vi "prova.vi"() -> ()   [LabVIEW 2025]
uses:
  <instrlib>/Keithley 2600 Series/Keithley 2600 Series.lvlib
panel:
  out "String 5":string
  out "String 4":string
  out "String 3":string
  out "String 2":string
  out "range misurato":string
  out "range misurato 2":string
  in  "source_range_gate":dbl format="%#_13g"
  in  "source_range_drain":dbl format="%#_13g"
  in  "dual sweep":bool
  out "error out":errorcluster
  in  "Boolean 4":bool
  in  "Boolean 3":bool
  in  "inverti smu":bool
  in  "Autozero Mode (2: Autozero Auto) 2":i32(ring)=2 items=["Autozero Off", "Autozero Once", "Autozero Auto"]
  in  "Autozero Mode (2: Autozero Auto)":i32(ring)=2 items=["Autozero Off", "Autozero Once", "Autozero Auto"]
  in  "Source Function (1: Voltage) 2":i32(ring)=1 items=["Current", "Voltage"]
  in  "Range Mode (1: Auto Range On) 2":i32(ring)=1 items=["Auto Range Off", "Auto Range On", "Auto Range Follow Limit"]
  in  "Source Function (1: Voltage)":i32(ring)=1 items=["Current", "Voltage"]
  in  "Range Mode (1: Auto Range On)":i32(ring)=1 items=["Auto Range Off", "Auto Range On", "Auto Range Follow Limit"]
  in  "range-gate":dbl format="%#_13g"
  in  "range-drain":dbl format="%#_13g"
  in  "limit-gate":dbl format="%#_13g"
  in  "limit-drain":dbl format="%#_13g"
  out "intervallo tra due misure approx (S)":dbl
  out "Frequenza di rete (Hz)":dbl
  in  "Numero di punti":i32
  out "finestra di misura (S)":dbl
  in  "Delay Time (S)":dbl
  in  "String":string
  in  "numero di sweep ripetute\n(piramidi per dual sweep)":i32
  in  "nplc":dbl
  in  "Boolean":bool
  in  "Pulse Stop Level (1 V) 2":dbl
  in  "Pulse Start Level (0 V) 2":dbl
  out "SMUB-TEMPI":dbl[](array[numeric])
  out "SMUB-TENSIONE":dbl[](array[numeric])
  out "SMUB-CORRENTE":dbl[](array[numeric])
  out "SMUA-TEMPI":dbl[](array[numeric])
  out "SMUA-TENSIONE":dbl[](array[numeric])
  out "SMUA-CORRENTE":dbl[](array[numeric])
  in  "stop 2":bool
  in  "stop":bool
  out "Firmware Revision":string
  out "Serial Number":string
  out "Model":string
  in  "VISA resource name":refnum<visa-resource-name>
  # "Impostazioni funzione source"
  # "Impostazioni connessione"
  # "DRAIN"
  # "GATE"
  # "Auto Range Off"
  # "Auto Range On"
  # "Auto Range Off"
  # "Auto Range On"
  # "non utilizzato...funzioni di lua per automatizzare il range"
  # "Impostazioni comuni"
  # "Impostazioni funzione misura"
  # "GATE"
  # "DRAIN"
  # "(1/"
  # "X"
  # ")"
  # "Auto Range Off"
  # "Auto Range On"
  # "Auto Range Off"
  # "Auto Range On"
  # "+"
  # "Controllo misura"
  # "tabella valori"
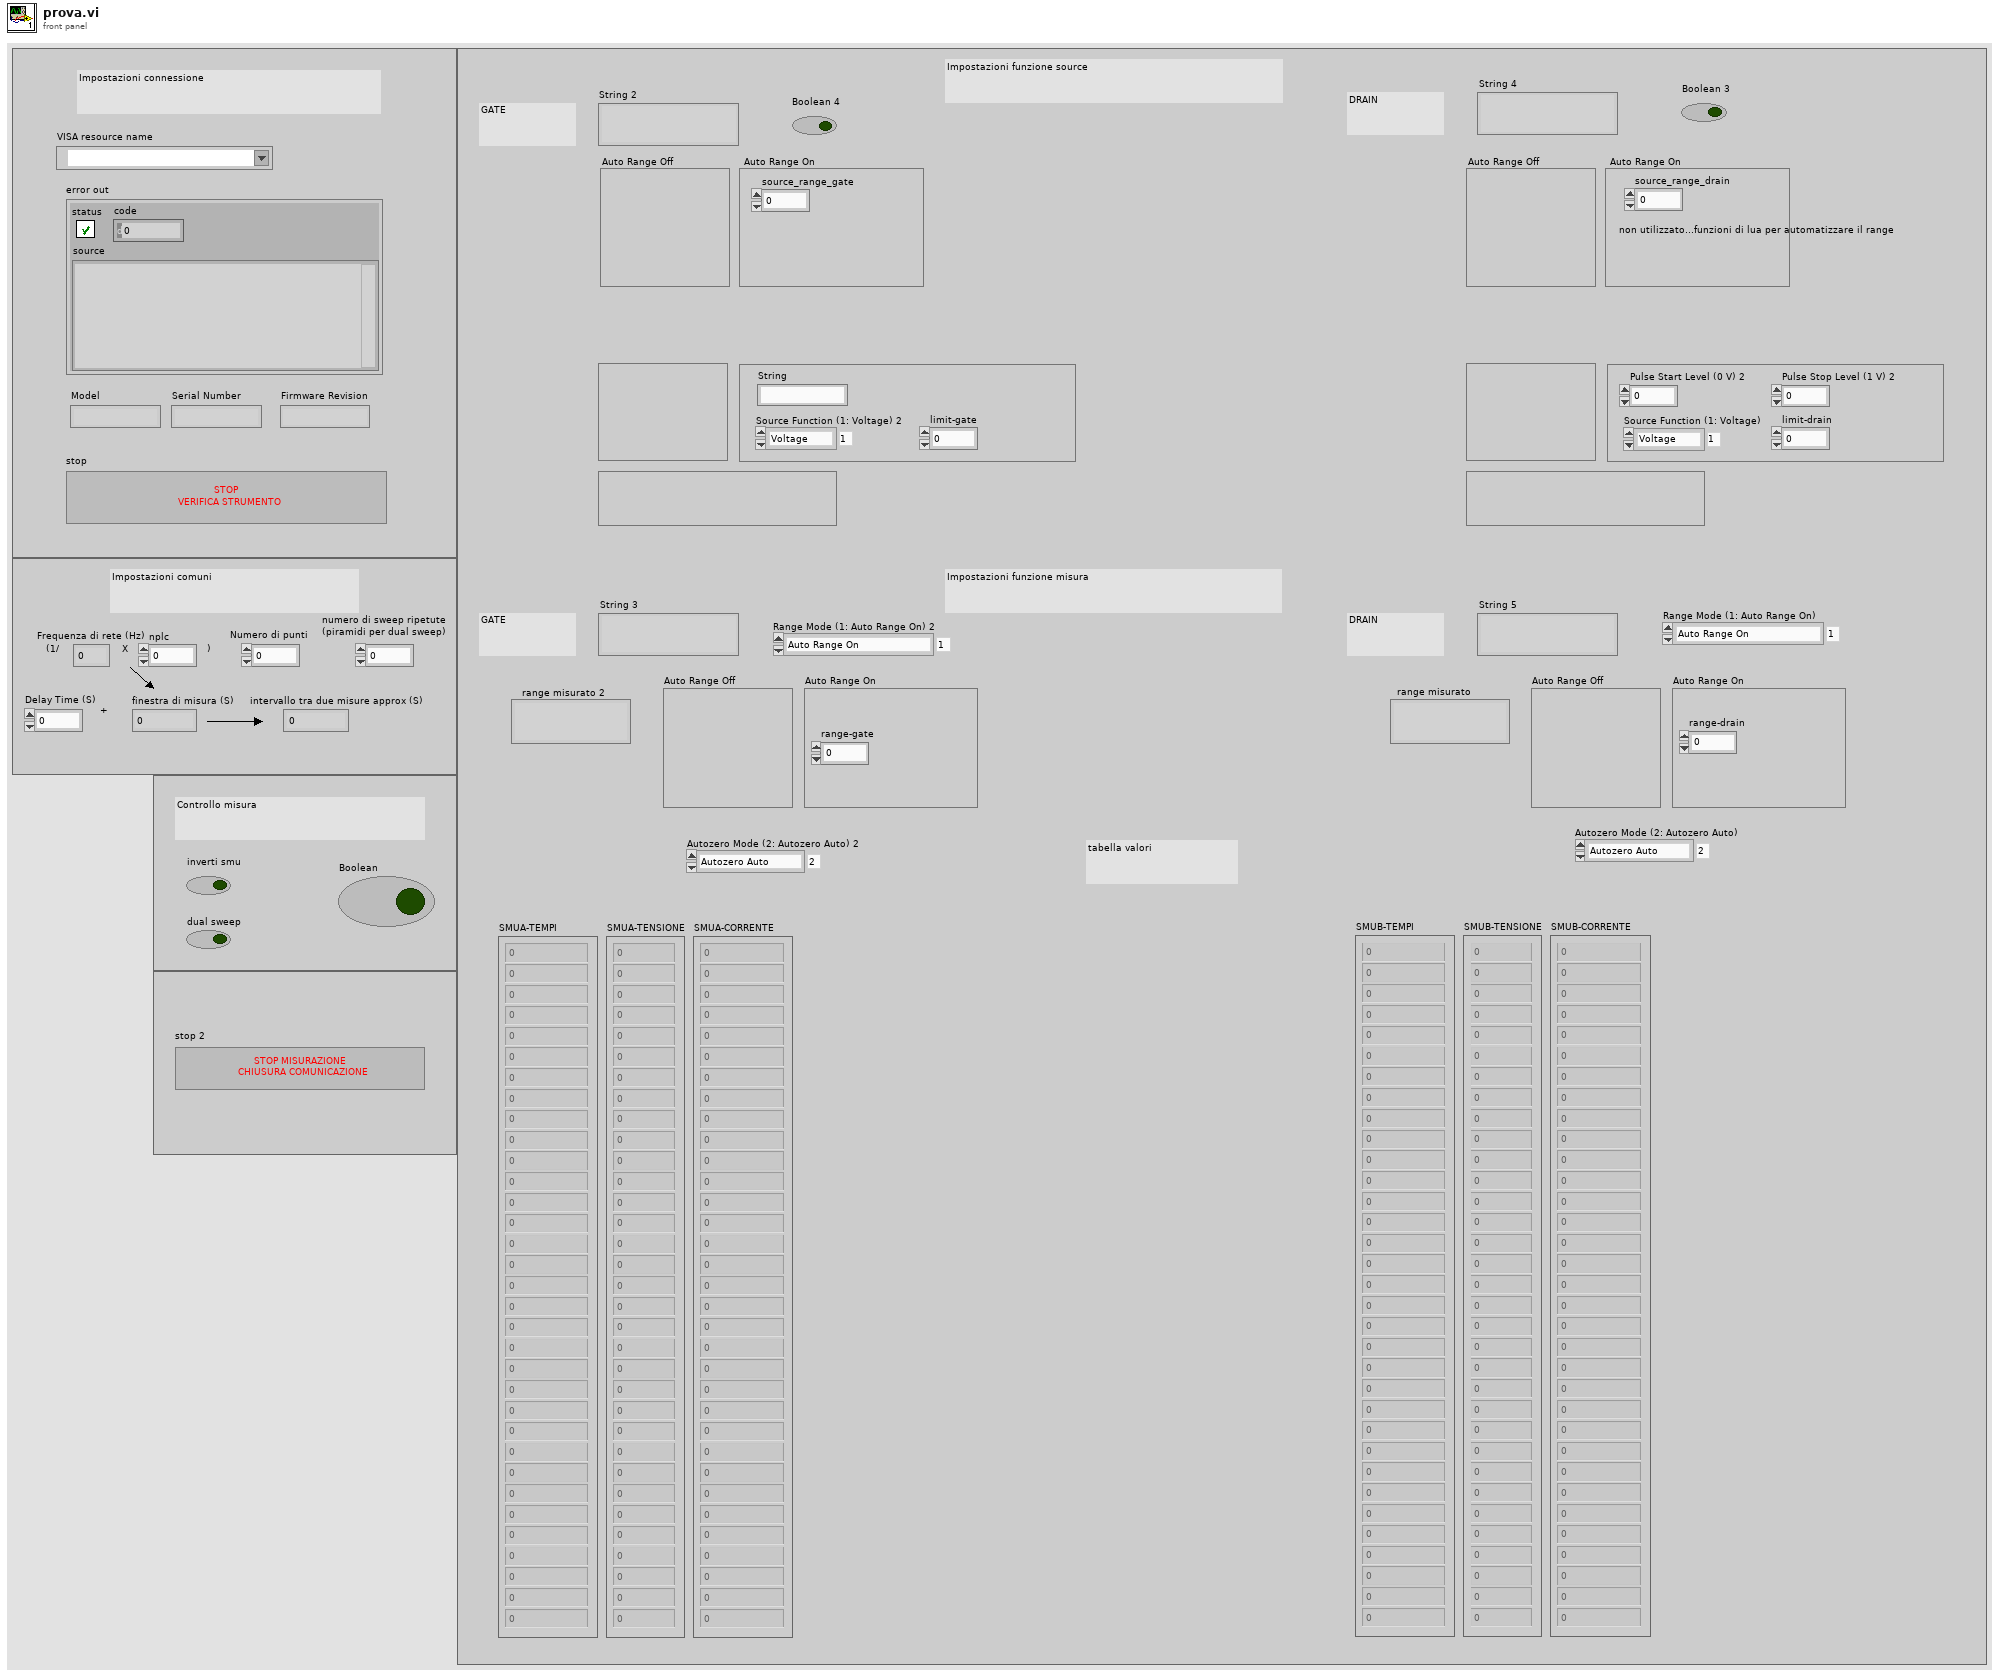
[diagram p1: front panel]
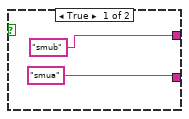
[diagram p2: hidden frame]
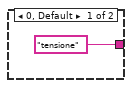
[diagram p3: hidden frame]
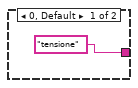
[diagram p4: hidden frame]
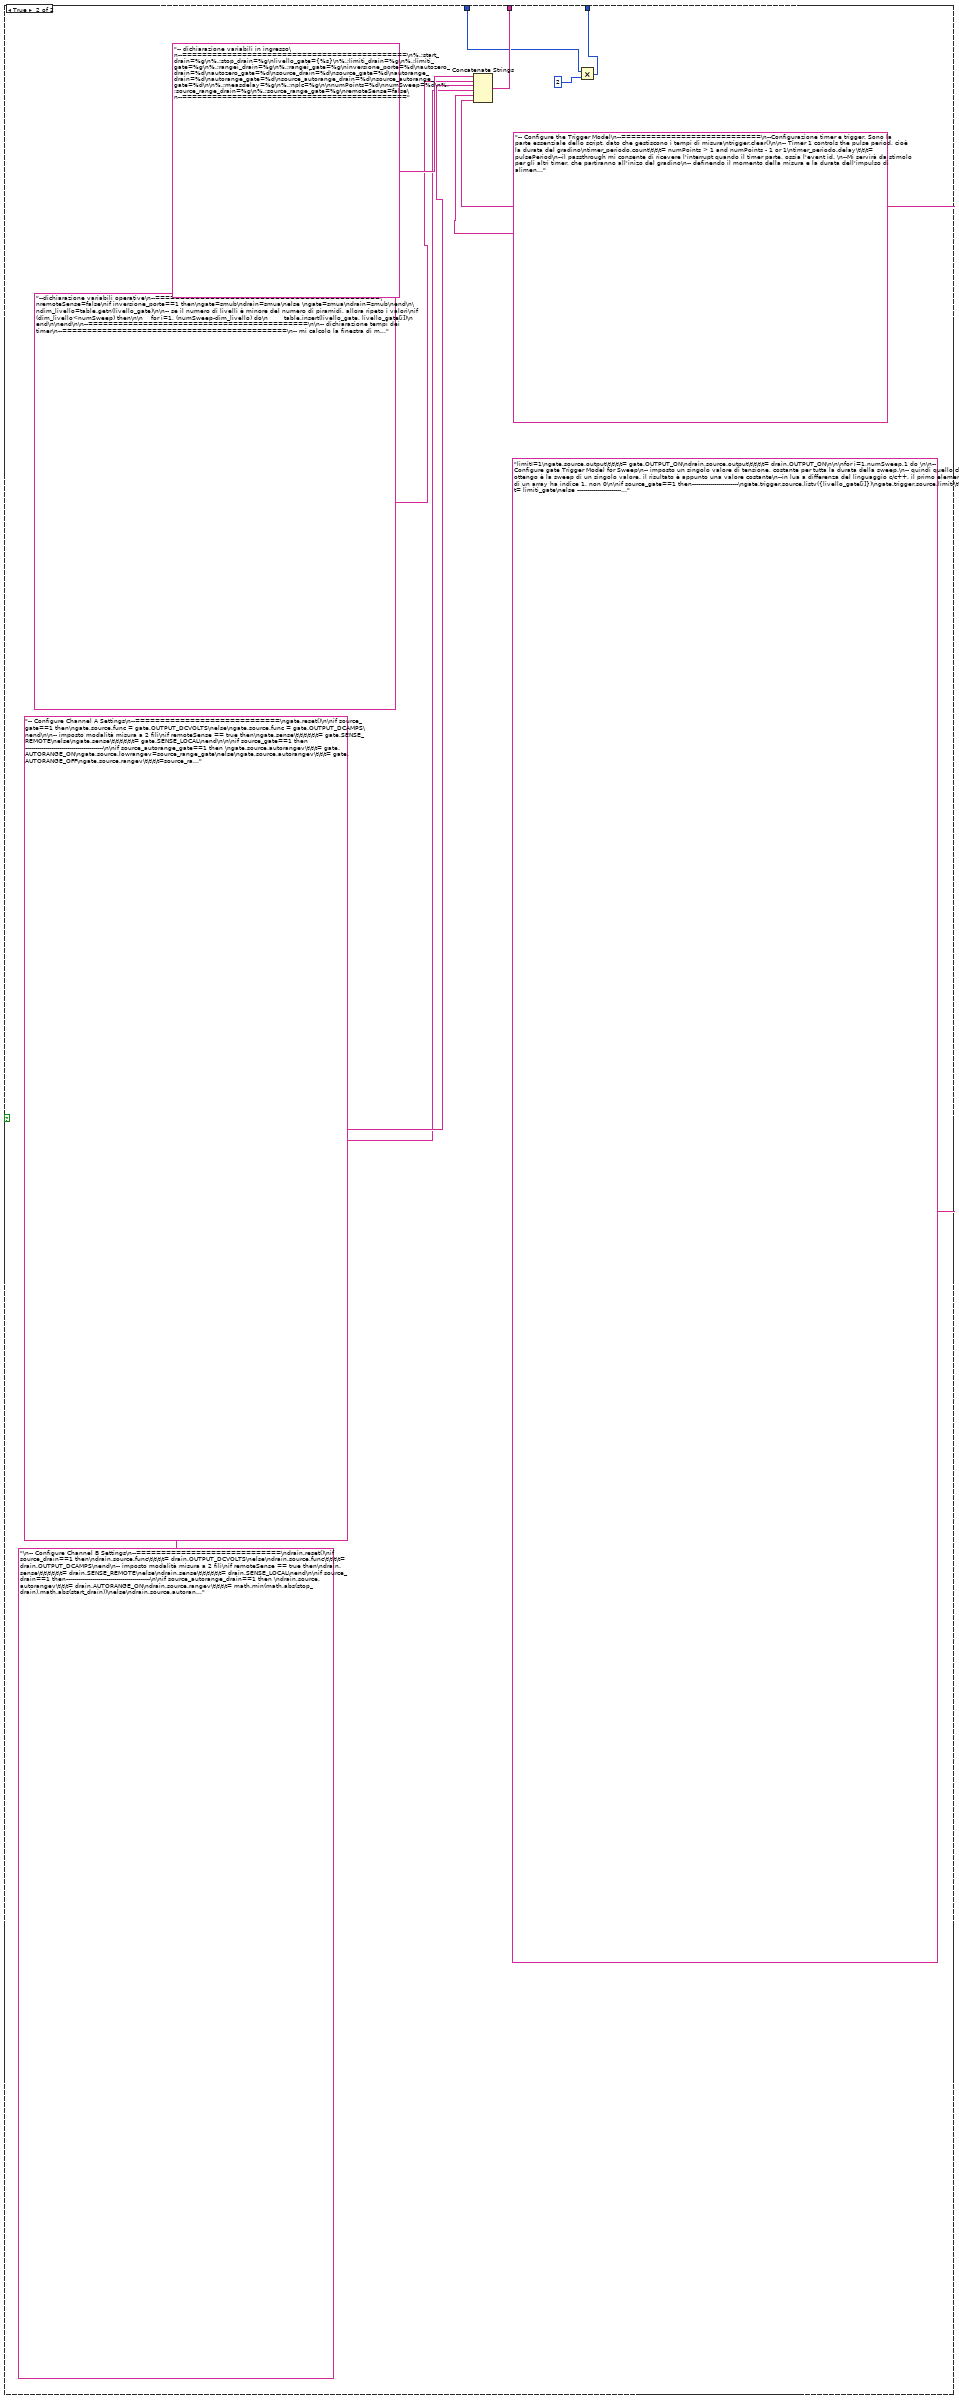
[diagram p6: hidden frame]
diagram:
  n1 = flat-sequence {
    tunnel: [w10] -> w5
    tunnel: [w7] -> w4
    tunnel: [w14] -> w6
    tunnel: w5 -> [w16]
    tunnel: w4 -> [w15]
    tunnel: [w13] -> w3
    tunnel: w6 -> [w28]
    tunnel: w3 -> [w27]
    tunnel: [w26] -> w2
    tunnel: [w25] -> w1
    tunnel: w2 -> [w147]
    tunnel: w1 -> [w146]
    frame #0 {
      w11 = "0\n\n"
      n2 = local write "Firmware Revision"(w11) -> ()
      n3 = local write "Serial Number"(w11) -> ()
      n4 = local write "Model"(w11) -> ()
      n5 = call <instrlib>:"Initialize.vi"("Reset (True)"=TRUE, "ID Query (True)"=FALSE, "VISA resource name"="VISA resource name") -> ("error out"=w7:errorcluster, "VISA resource name out"=w10:refnum<visa-resource-name>)  [unwired: 7 in]
      "error out" <- w7
    }
    frame #1 {
      n6 = while {
        tunnel: w16 -> [w20]
        tunnel: w15 -> [w19]
        tunnel: [w18] -> w14
        tunnel: [w17] -> w13
        stop <- "stop" stop-if-true
        n7 = call <instrlib>:"Query Local Node Identity.vi"("error in (no error)"=w19, "VISA resource name"=w20) -> ("error out"=w17:errorcluster, "Serial Number"=→"Serial Number":string, "Model"=→"Model":string, "VISA resource name out"=w18:refnum<visa-resource-name>, "Firmware Revision"=→"Firmware Revision":string)  [unwired: 5 in]
      }
    }
    frame #2 {
      n8 = while {
        tunnel: w28 -> [w53]
        tunnel: w27 -> [w52]
        tunnel: [w68] -> w26
        tunnel: [w67] -> w25
        stop <- "stop 2" stop-if-true
        n9 = case shown="False" "inverti smu" {
          tunnel: ["smub" "smua"] -> w31
          tunnel: ["smua" "smub"] -> w30
          frame True {
          }
          frame False {
          }
        }
        "String 2" <- w31
        "String 3" <- w31
        "String 4" <- w30
        "String 5" <- w30
        n10 = call <instrlib>:"Print Variable.vi"("error in (no error)"=w52, "Variable Name"="localnode.linefreq", "VISA resource name"=w53) -> ("error out"=w50:errorcluster, "Number"=w57:dbl, "VISA resource name out"=w51:refnum<visa-resource-name>)  [unwired: 5 in, 1 out]
        "Frequenza di rete (Hz)" <- w57
        n11 = Divide(x=1.0, y=w57) -> (x/y=w62:dbl)
        n12 = Multiply(x="nplc", y=w62) -> (x*y=w54:dbl)
        "finestra di misura (S)" <- w54
        n13 = Add(x="Delay Time (S)", y=w54) -> (x+y=→"intervallo tra due misure approx (S)":dbl)
        n14 = case shown="1" "Source Function (1: Voltage) 2" {
          tunnel: ["tensione" "corrente"] -> w34
          frame 0, Default {
          }
          frame 1 {
          }
        }
        "range misurato" <- w34
        n15 = case shown="1" "Source Function (1: Voltage)" {
          tunnel: ["tensione" "corrente"] -> w35
          frame 0, Default {
          }
          frame 1 {
          }
        }
        "range misurato 2" <- w35
        n16 = case shown="True" "Boolean" {
          tunnel: [w79 w114] -> w68
          tunnel: [w78 w113] -> w67
          tunnel: w50 -> [w78 w123]
          tunnel: w51 -> [w79 w124]
          tunnel: "Pulse Start Level (0 V) 2" -> [_ w104]
          tunnel: "Pulse Stop Level (1 V) 2" -> [_ w103]
          tunnel: "Numero di punti" -> [_ w85]
          tunnel: "Delay Time (S)" -> [_ w89]
          tunnel: "numero di sweep ripetute\n(piramidi per dual sweep)" -> [_ w84]
          tunnel: "String" -> [_ w102]
          tunnel: "limit-drain" -> [_ w101]
          tunnel: "limit-gate" -> [_ w100]
          tunnel: "range-drain" -> [_ w99]
          tunnel: "range-gate" -> [_ w98]
          tunnel: "inverti smu" -> [_ w97]
          tunnel: "Autozero Mode (2: Autozero Auto)" -> [_ w96]
          tunnel: "Autozero Mode (2: Autozero Auto) 2" -> [_ w95]
          tunnel: "Source Function (1: Voltage)" -> [_ w94]
          tunnel: "Source Function (1: Voltage) 2" -> [_ w93]
          tunnel: "Range Mode (1: Auto Range On)" -> [_ w92]
          tunnel: "Range Mode (1: Auto Range On) 2" -> [_ w91]
          tunnel: "nplc" -> [_ w90]
          tunnel: "Boolean 3" -> [_ w88]
          tunnel: "Boolean 4" -> [_ w87]
          tunnel: "dual sweep" -> [_ w86]
          tunnel: "source_range_drain" -> [_ w81]
          tunnel: "source_range_gate" -> [_ w80]
          frame False {
          }
          frame True {
            w112 = 0 items=["Channel A", "Channel B"] ("Source Measure Unit Channel (0: Channel A)")
            w115 = 1 items=["Channel A", "Channel B"] ("Source Measure Unit Channel (0: Channel A)")
            n17 = Multiply(x=w85, y=w84) -> (x*y=w83:i32)
            n18 = case shown="False" w86 {
              tunnel: [w128 w139] -> w105
              tunnel: w83 -> [w127 w137]
              tunnel: [w126 w138] -> w82
              frame False {
                n19 = Concatenate Strings("-- dichiarazione variabili in ingresso\n--=============================================\n%.;start_drain=%g\n%.;stop_drain=%g\nlivello_gate={%s}\n%.;limiti_drain=%g\n%.;limiti_gate=%g\n%.;rangei_drain=%g\n%.;rangei_gate=%g\ninversione_porte=%d\nautozero_drain=%d\nautozero_gate=%d\nsource_drain=%d\nsource_gate=%d\nautorange_drain=%d\nautorange_gate=%d\nsource_autorange_drain=%d\nsource_autorange_gate=%d\n\n%.;measdelay=%g\n%.;nplc=%g\n\nnumPoints=%d\nnumSweep=%d\nremoteSense=false\n%.;source_range_drain=%g\n%.;source_range_gate=%g\n--=============================================", "--dichiarazione variabili operative\n--=============================================\nremoteSense=false\nif inversione_porte==1 then\ngate=smub\ndrain=smua\nelse \ngate=smua\ndrain=smub\nend\n--============================================\n\n-- dichiarazione tempi dei timer\n--=============================================\n-- mi calcolo la finestra di misura\nfinestra_misura=(1/localnode.linefreq)*nplc\n-- imposto la lunghezza dell'impulso. la dc sweep si origina da una pulsed sweep.\npulseWidth=measdelay+finestra_misura \n--il periodo è l'impulso + più un t_off, una bassa percentuale dell'impulso\npulsePeriod=pulseWidth+(pulseWidth*1/100) \n\n--=============================================\n\n-- dichiarazione timer e gestore eventi\n--=============================================\n-- Timer 1: timer periodo (larghezza gradino)\ntimer_periodo=trigger.timer[1]\n-- Timer 2: Timer ritardo misura\ntimer_misura=trigger.timer[2]\n-- Timer 3: Pulse Width Timer\ntimer_larghezza_impulso=trigger.timer[3]\n\n-- Gestore eventi 1: Event Blender per la partenza di iniziale di smua e l'aggiornamento di smua al trigger di smub\ngestore_avvio_gate=trigger.blender[1]\n--=============================================", "-- Configure Channel A Settings\n--=============================\ngate.reset()\n\nif source_gate==1 then\ngate.source.func = gate.OUTPUT_DCVOLTS\nelse\ngate.source.func = gate.OUTPUT_DCAMPS\nend\n\n-- imposto modalità misura a 2 fili\nif remoteSense == true then\ngate.sense\t\t\t\t\t\t= gate.SENSE_REMOTE\nelse\ngate.sense\t\t\t\t\t\t= gate.SENSE_LOCAL\nend\n\n\nif source_gate==1 then ---------------------------------------\n\nif source_autorange_gate==1 then \ngate.source.autorangev\t\t\t= gate.AUTORANGE_ON\ngate.source.lowrangev= source_range_gate\nelse\ngate.source.autorangev\t\t\t= gate.AUTORANGE_OFF\ngate.source.rangev\t\t\t\t= source_range_gate\nend \n\ngate.source.levelv\t\t\t\t= 0\n-- Set the DC bias limit.  This is not the limit used during the pulses. ma è il valore di idle della gate\ngate.source.limiti\t\t\t\t= limiti_gate\n\nelse------------------------\n\nif source_autorange_gate==1 then\ngate.source.autorangei\t\t\t= gate.AUTORANGE_ON\ngate.source.lowrangei=source_range_gate\nelse\ngate.source.autorangei\t\t\t= gate.AUTORANGE_OFF\ngate.source.rangei\t\t\t=source_range_gate\nend\n\ngate.source.leveli\t\t\t\t= 0\n-- Set the DC bias limit.  This is not the limit used during the pulses. ma è il valore di idle della gate\ngate.source.limitv\t\t\t\t= limiti_gate\nend --------------------------------------------------\n\n\n-- Disabling Auto-Ranging and Auto-Zero ensures accurate and consistent timing\nif autozero_gate==0 then\ngate.measure.autozero\t\t\t= gate.AUTOZERO_OFF\nelseif autozero_gate==1 then\ngate.measure.autozero\t\t\t= gate.AUTOZERO_ONCE\nelse\ngate.measure.autozero\t\t\t= gate.AUTOZERO_AUTO\nend\n\nif autorange_gate==0 then ------------------------\n\nif source_gate==1 then\ngate.measure.autorangei\t\t\t= gate.AUTORANGE_OFF\ngate.measure.rangei\t\t\t\t= rangei_gate\nelse\ngate.measure.autorangev\t\t\t= gate.AUTORANGE_OFF\ngate.measure.rangev\t\t\t\t= rangei_gate\nend\n\nelseif  autorange_gate==1 then -----------\n\nif source_gate==1 then\ngate.measure.autorangei\t\t\t= gate.AUTORANGE_ON\ngate.measure.lowrangei\t\t\t\t= rangei_gate\nelse\ngate.measure.autorangev\t\t\t= gate.AUTORANGE_ON\ngate.measure.lowrangev\t\t\t\t= rangei_gate\nend\n\nelse --------------------------\n\nend -------------------------------\n\ngate.measure.nplc\t\t\t\t= nplc\n-- A timer will be used to set the measure delay and synchronize the measurement\n-- between the two SMUs so set the built in delay to 0.\ngate.measure.delay\t\t\t\t= 0\n\n-- Prepare the Reading Buffers\ngate.nvbuffer1.clear()\ngate.nvbuffer1.collecttimestamps= 1\ngate.nvbuffer2.clear()\ngate.nvbuffer2.collecttimestamps = 1\n--=============================\n-- End Channel A Settings", "\n-- Configure Channel B Settings\n--=============================\ndrain.reset()\nif source_drain==1 then\ndrain.source.func\t\t\t\t= drain.OUTPUT_DCVOLTS\nelse\ndrain.source.func\t\t\t\t= drain.OUTPUT_DCAMPS\nend\n-- imposto modalità misura a 2 fili\nif remoteSense == true then\ndrain.sense\t\t\t\t\t\t= drain.SENSE_REMOTE\nelse\ndrain.sense\t\t\t\t\t\t= drain.SENSE_LOCAL\nend\n\nif source_drain==1 then------------------------------------------\n\nif source_autorange_drain==1 then \ndrain.source.autorangev\t\t\t= drain.AUTORANGE_ON\ndrain.source.rangev\t\t\t\t= math.min(math.abs(stop_drain),math.abs(start_drain))\nelse\ndrain.source.autorangev\t\t\t= drain.AUTORANGE_OFF\ndrain.source.rangev\t\t\t\t=  math.max(math.abs(stop_drain),math.abs(start_drain))\nend\n\ndrain.source.levelv\t\t\t\t= 0\n-- Set the DC bias limit.  This is not the limit used during the pulses. ma è il valore di idle della smu\ndrain.source.limiti\t\t\t\t= limiti_drain\nelse----------------------------------------------------\nif source_autorange_drain==1 then \ndrain.source.autorangei\t\t\t= drain.AUTORANGE_ON\ndrain.source.rangei\t\t\t\t= math.min(math.abs(stop_drain),math.abs(start_drain))\nelse\ndrain.source.autorangei\t\t\t= drain.AUTORANGE_OFF\ndrain.source.rangei\t\t\t\t= math.max(math.abs(stop_drain),math.abs(start_drain))\nend\ndrain.source.leveli\t\t\t\t= 0\n-- Set the DC bias limit.  This is not the limit used during the pulses. ma è il valore di idle della smu\ndrain.source.limitv\t\t\t\t= limiti_drain\nend----------------------------------------------\n\n-- Disabling Auto-Ranging and Auto-Zero ensures accurate and consistent timing\n\nif autozero_drain==0 then\ndrain.measure.autozero\t\t\t= drain.AUTOZERO_OFF\nelseif autozero_drain==1 then\ndrain.measure.autozero\t\t\t= drain.AUTOZERO_ONCE\nelseif autozero_drain==2 then\ndrain.measure.autozero\t\t\t= drain.AUTOZERO_AUTO\nend\n\nif autorange_drain==0 then --------------------------------\n\nif source_drain==1 then\ndrain.measure.autorangei\t\t\t= drain.AUTORANGE_OFF\ndrain.measure.rangei\t\t\t\t= rangei_drain\nelse\ndrain.measure.autorangev\t\t\t= drain.AUTORANGE_OFF\ndrain.measure.rangev\t\t\t\t= rangei_drain\nend\n\n\n\nelseif  autorange_drain==1 then ----------------------------\n\nif source_drain==1 then\ndrain.measure.autorangei\t\t\t= drain.AUTORANGE_ON\ndrain.measure.lowrangei\t\t\t\t= rangei_drain\nelse\ndrain.measure.autorangev\t\t\t= drain.AUTORANGE_ON\ndrain.measure.lowrangev\t\t\t\t= rangei_drain\nend\n\nelse\n\nend --------------------------------------------------------------\n\ndrain.measure.nplc\t\t\t\t= nplc\n-- A timer will be used to set the measure delay and synchronize the measurement\n-- between the two SMUs so set the built in delay to 0.\ndrain.measure.delay\t\t\t\t= 0\n\n-- Prepare the Reading Buffers\ndrain.nvbuffer1.clear()\ndrain.nvbuffer1.collecttimestamps= 1\ndrain.nvbuffer2.clear()\ndrain.nvbuffer2.collecttimestamps= 1\n--=============================\n-- End Channel B Settings", "-- Configure the Trigger Model\n--============================\n--Configurazione timer e trigger. Sono la parte essenziale dello script, dato che gestiscono i tempi di misura\ntrigger.clear()\n\n-- Timer 1 controls the pulse period, cioè la durata del gradino\ntimer_periodo.count\t\t\t= numPoints > 1 and numPoints - 1 or 1\ntimer_periodo.delay\t\t\t= pulsePeriod\n--il passthrough mi consente di ricevere l'interrupt quando il timer parte, ossia l'event id. \n--Mi servirà da stimolo per gli altri timer, che partiranno all'inizo del gradino\n-- definendo il momento della misura e la durata dell'impulso di alimentazione\ntimer_periodo.passthrough\t= true\n-- il timer 1 parte quando la drain, in questo caso, inizia la sweep: cioè entra nello stato armed\ntimer_periodo.stimulus\t\t= drain.trigger.ARMED_EVENT_ID \n\n-- Timer 2 controls the measurement. il timer 2 gestisce il ritardo di misura. scaduto quello, inizia la finestra di misura\ntimer_misura.count\t\t\t= 1\ntimer_misura.delay\t\t\t= measdelay\n-- il passthrough è false perchè l'interrupt lo produrre alla fine. \n-- Scaduto il delay di misura, inizia la finestra di misura\ntimer_misura.passthrough\t= false\n--il timer 1 grazie al passthrough mi fa partire il timer 2 all'inizio del gradino\ntimer_misura.stimulus\t\t= timer_periodo.EVENT_ID \n\n-- Timer 3 controls the pulse width\ntimer_larghezza_impulso.count\t\t\t= 1\ntimer_larghezza_impulso.delay\t\t\t= pulseWidth\n-- il passthrough è false perchè l'interrupt me lo produce alla fine, perchè \ntimer_larghezza_impulso.passthrough\t= false\n--il timer 1 grazie al passthrough mi fa partire il timer 3 all'inizio del gradino\ntimer_larghezza_impulso.stimulus\t\t= timer_periodo.EVENT_ID\n", "\n-- Configure gate Trigger Model for Sweep\n-- imposto un singolo valore di tensione, costante per tutta la durata della sweep.\n-- quindi quello che ottengo è la sweep di un singolo valore. il risultato è appunto una valore costante\nif source_gate==1 then-----------------------\ngate.trigger.source.listv(livello_gate)\ngate.trigger.source.limiti\t\t= limiti_gate\nelse -------------------------------------------\ngate.trigger.source.listi(livello_gate)\ngate.trigger.source.limitv\t\t= limiti_gate\nend--------------------------------------------\ngate.trigger.measure.action\t\t= gate.ASYNC\ngate.trigger.measure.iv(gate.nvbuffer1, gate.nvbuffer2)\n--fine impulso: se voglio una dc sweep, anzichè mandare in idle l'uscita, la tengo costante\ngate.trigger.endpulse.action\t= gate.SOURCE_HOLD\n-- endsweep mi dice cosa fare quando finisce l'operazione sweep\ngate.trigger.endsweep.action\t= gate.SOURCE_HOLD\ngate.trigger.arm.count = 1\ngate.trigger.count\t\t\t\t= numSweep\n-- arm sweep indica quanto sweep deve fare \ndrain.trigger.arm.stimulus\t\t= 0\n\n\n--event blender per la partenza\ngestore_avvio_gate.orenable = true\ngestore_avvio_gate.stimulus[1] = gate.trigger.ARMED_EVENT_ID\ngestore_avvio_gate.stimulus[2] = drain.trigger.ARMED_EVENT_ID \n\n--dico quali stimoli/timer attivano le azioni\ngate.trigger.source.stimulus = gestore_avvio_gate.EVENT_ID \ngate.trigger.measure.stimulus\t= timer_misura.EVENT_ID\ngate.trigger.endpulse.stimulus\t= drain.trigger.SWEEP_COMPLETE_EVENT_ID\n\ngate.trigger.source.action\t\t= gate.ENABLE\n\n-- Configure drain Trigger Model for Sweep\nif source_drain==1 then------------------------\ndrain.trigger.source.linearv(start_drain, stop_drain, numPoints)\ndrain.trigger.source.limiti\t\t= limiti_drain\nelse---------------------------------------------\ndrain.trigger.source.lineari(start_drain, stop_drain, numPoints)\ndrain.trigger.source.limitv\t\t= limiti_drain\nend---------------------------------------------\ndrain.trigger.measure.action\t\t= drain.ENABLE\ndrain.trigger.measure.iv(drain.nvbuffer1, drain.nvbuffer2)\n--fine impulso: se voglio una dc sweep, anzichè mandare in idle l'uscita, la tengo costante\ndrain.trigger.endpulse.action\t= drain.SOURCE_HOLD \n-- endsweep mi dice cosa fare quando finisce l'operazione sweep\ndrain.trigger.endsweep.action\t= drain.SOURCE_HOLD\ndrain.trigger.arm.count = numSweep\n-- num punti sweep\ndrain.trigger.count\t\t\t\t= numPoints\n-- arm sweep indica quanto sweep deve fare\ndrain.trigger.arm.stimulus\t\t= 0\n--dico quali timer attivanzo le azioni\ndrain.trigger.source.stimulus\t= timer_periodo.EVENT_ID\ndrain.trigger.measure.stimulus\t= timer_misura.EVENT_ID\ndrain.trigger.endpulse.stimulus\t= timer_larghezza_impulso.EVENT_ID\ndrain.trigger.source.action\t\t= drain.ENABLE\n--==============================\n-- End Trigger Model Configuration" ("write buffer"), "\ngate.source.output\t\t\t\t= gate.OUTPUT_ON\ndrain.source.output\t\t\t\t= drain.OUTPUT_ON\n\n-- Start the trigger model execution\ngate.trigger.initiate()\ndelay(0.05)\ndrain.trigger.initiate()\n\n-- Wait until the sweep has completed\nwaitcomplete()\n\ndrain.source.output\t\t\t\t= drain.OUTPUT_OFF\ndelay(0.05)\ngate.source.output\t\t\t\t= gate.OUTPUT_OFF\n\n--printbuffer(1, numPoints, gate.nvbuffer2.readings)\n--printbuffer(1, numPoints, gate.nvbuffer1.readings)\n--printbuffer(1, numPoints, gate.nvbuffer1.timestamps)\n\n--printbuffer(1, numPoints, drain.nvbuffer2.readings)\n--printbuffer(1, numPoints, drain.nvbuffer1.readings)\n--printbuffer(1, numPoints, drain.nvbuffer1.timestamps)\n") -> (w128:string)
                n20 = Multiply(x=w127, y=1) -> (x*y=w126:i32)
              }
              frame True {
                n21 = Concatenate Strings("-- dichiarazione variabili in ingresso\n--=============================================\n%.;start_drain=%g\n%.;stop_drain=%g\nlivello_gate={%s}\n%.;limiti_drain=%g\n%.;limiti_gate=%g\n%.;rangei_drain=%g\n%.;rangei_gate=%g\ninversione_porte=%d\nautozero_drain=%d\nautozero_gate=%d\nsource_drain=%d\nsource_gate=%d\nautorange_drain=%d\nautorange_gate=%d\nsource_autorange_drain=%d\nsource_autorange_gate=%d\n\n%.;measdelay=%g\n%.;nplc=%g\n\nnumPoints=%d\nnumSweep=%d\n%.;source_range_drain=%g\n%.;source_range_gate=%g\nremoteSense=false\n--=============================================", "--dichiarazione variabili operative\n--=============================================\nremoteSense=false\nif inversione_porte==1 then\ngate=smub\ndrain=smua\nelse \ngate=smua\ndrain=smub\nend\n\ndim_livello=table.getn(livello_gate)\n\n-- se il numero di livelli è minore del numero di piramidi, allora ripeto i valori\nif (dim_livello<numSweep) then\n\n    for i=1, (numSweep-dim_livello) do\n        table.insert(livello_gate, livello_gate[i])\n    end\n\nend\n\n--============================================\n\n-- dichiarazione tempi dei timer\n--=============================================\n-- mi calcolo la finestra di misura\nfinestra_misura=(1/localnode.linefreq)*nplc\n-- imposto la lunghezza dell'impulso. la dc sweep si origina da una pulsed sweep.\npulseWidth=measdelay+finestra_misura \n--il periodo è l'impulso + più un t_off, una bassa percentuale dell'impulso\npulsePeriod=pulseWidth+(pulseWidth*1/100) \n--=============================================\n\n-- dichiarazione timer e gestore eventi\n--=============================================\n-- Timer 1: timer periodo (larghezza gradino)\ntimer_periodo=trigger.timer[1]\n-- Timer 2: Timer ritardo misura\ntimer_misura=trigger.timer[2]\n-- Timer 3: Pulse Width Timer\ntimer_larghezza_impulso=trigger.timer[3]\n\n-- Gestore eventi 1: Event Blender per la partenza di iniziale di smua e l'aggiornamento di smua al trigger di smub\ngestore_avvio_gate=trigger.blender[1]\n--=============================================", "-- Configure Channel A Settings\n--=============================\ngate.reset()\n\nif source_gate==1 then\ngate.source.func = gate.OUTPUT_DCVOLTS\nelse\ngate.source.func = gate.OUTPUT_DCAMPS\nend\n\n-- imposto modalità misura a 2 fili\nif remoteSense == true then\ngate.sense\t\t\t\t\t\t= gate.SENSE_REMOTE\nelse\ngate.sense\t\t\t\t\t\t= gate.SENSE_LOCAL\nend\n\n\nif source_gate==1 then ---------------------------------------\n\nif source_autorange_gate==1 then \ngate.source.autorangev\t\t\t= gate.AUTORANGE_ON\ngate.source.lowrangev=source_range_gate\nelse\ngate.source.autorangev\t\t\t= gate.AUTORANGE_OFF\ngate.source.rangev\t\t\t\t=source_range_gate\nend \n\ngate.source.levelv\t\t\t\t= 0\n-- Set the DC bias limit.  This is not the limit used during the pulses. ma è il valore di idle della gate\ngate.source.limiti\t\t\t\t= limiti_gate\n\nelse------------------------\n\nif source_autorange_gate==1 then\ngate.source.autorangei\t\t\t= gate.AUTORANGE_ON\ngate.source.lowrangei=source_range_gate\nelse\ngate.source.autorangei\t\t\t= gate.AUTORANGE_OFF\ngate.source.rangei\t\t\t=source_range_gate\nend\n\ngate.source.leveli\t\t\t\t= 0\n-- Set the DC bias limit.  This is not the limit used during the pulses. ma è il valore di idle della gate\ngate.source.limitv\t\t\t\t= limiti_gate\nend --------------------------------------------------\n\n\n-- Disabling Auto-Ranging and Auto-Zero ensures accurate and consistent timing\nif autozero_gate==0 then\ngate.measure.autozero\t\t\t= gate.AUTOZERO_OFF\nelseif autozero_gate==1 then\ngate.measure.autozero\t\t\t= gate.AUTOZERO_ONCE\nelse\ngate.measure.autozero\t\t\t= gate.AUTOZERO_AUTO\nend\n\nif autorange_gate==0 then ------------------------\n\nif source_gate==1 then\ngate.measure.autorangei\t\t\t= gate.AUTORANGE_OFF\ngate.measure.rangei\t\t\t\t= rangei_gate\nelse\ngate.measure.autorangev\t\t\t= gate.AUTORANGE_OFF\ngate.measure.rangev\t\t\t\t= rangei_gate\nend\n\nelseif  autorange_gate==1 then -----------\n\nif source_gate==1 then\ngate.measure.autorangei\t\t\t= gate.AUTORANGE_ON\ngate.measure.lowrangei\t\t\t\t= rangei_gate\nelse\ngate.measure.autorangev\t\t\t= gate.AUTORANGE_ON\ngate.measure.lowrangev\t\t\t\t= rangei_gate\nend\n\nelse --------------------------\n\nend -------------------------------\n\ngate.measure.nplc\t\t\t\t= nplc\n-- A timer will be used to set the measure delay and synchronize the measurement\n-- between the two SMUs so set the built in delay to 0.\ngate.measure.delay\t\t\t\t= 0\n\n-- Prepare the Reading Buffers\ngate.nvbuffer1.clear()\ngate.nvbuffer1.collecttimestamps= 1\ngate.nvbuffer1.appendmode=1\ngate.nvbuffer2.clear()\ngate.nvbuffer2.collecttimestamps = 1\ngate.nvbuffer2.appendmode=1\n--=============================\n-- End Channel A Settings", "\n-- Configure Channel B Settings\n--=============================\ndrain.reset()\nif source_drain==1 then\ndrain.source.func\t\t\t\t= drain.OUTPUT_DCVOLTS\nelse\ndrain.source.func\t\t\t\t= drain.OUTPUT_DCAMPS\nend\n-- imposto modalità misura a 2 fili\nif remoteSense == true then\ndrain.sense\t\t\t\t\t\t= drain.SENSE_REMOTE\nelse\ndrain.sense\t\t\t\t\t\t= drain.SENSE_LOCAL\nend\n\nif source_drain==1 then------------------------------------------\n\nif source_autorange_drain==1 then \ndrain.source.autorangev\t\t\t= drain.AUTORANGE_ON\ndrain.source.rangev\t\t\t\t= math.min(math.abs(stop_drain),math.abs(start_drain))\nelse\ndrain.source.autorangev\t\t\t= drain.AUTORANGE_OFF\ndrain.source.rangev\t\t\t\t=  math.max(math.abs(stop_drain),math.abs(start_drain))\nend\n\ndrain.source.levelv\t\t\t\t= 0\n-- Set the DC bias limit.  This is not the limit used during the pulses. ma è il valore di idle della smu\ndrain.source.limiti\t\t\t\t= limiti_drain\nelse----------------------------------------------------\nif source_autorange_drain==1 then \ndrain.source.autorangei\t\t\t= drain.AUTORANGE_ON\ndrain.source.rangei\t\t\t\t= math.min(math.abs(stop_drain),math.abs(start_drain))\nelse\ndrain.source.autorangei\t\t\t= drain.AUTORANGE_OFF\ndrain.source.rangei\t\t\t\t= math.max(math.abs(stop_drain),math.abs(start_drain))\nend\ndrain.source.leveli\t\t\t\t= 0\n-- Set the DC bias limit.  This is not the limit used during the pulses. ma è il valore di idle della smu\ndrain.source.limitv\t\t\t\t= limiti_drain\nend----------------------------------------------\n\n-- Disabling Auto-Ranging and Auto-Zero ensures accurate and consistent timing\n\nif autozero_drain==0 then\ndrain.measure.autozero\t\t\t= drain.AUTOZERO_OFF\nelseif autozero_drain==1 then\ndrain.measure.autozero\t\t\t= drain.AUTOZERO_ONCE\nelseif autozero_drain==2 then\ndrain.measure.autozero\t\t\t= drain.AUTOZERO_AUTO\nend\n\nif autorange_drain==0 then --------------------------------\n\nif source_drain==1 then\ndrain.measure.autorangei\t\t\t= drain.AUTORANGE_OFF\ndrain.measure.rangei\t\t\t\t= rangei_drain\nelse\ndrain.measure.autorangev\t\t\t= drain.AUTORANGE_OFF\ndrain.measure.rangev\t\t\t\t= rangei_drain\nend\n\n\n\nelseif  autorange_drain==1 then ----------------------------\n\nif source_drain==1 then\ndrain.measure.autorangei\t\t\t= drain.AUTORANGE_ON\ndrain.measure.lowrangei\t\t\t\t= rangei_drain\nelse\ndrain.measure.autorangev\t\t\t= drain.AUTORANGE_ON\ndrain.measure.lowrangev\t\t\t\t= rangei_drain\nend\n\nelse\n\nend --------------------------------------------------------------\n\ndrain.measure.nplc\t\t\t\t= nplc\n-- A timer will be used to set the measure delay and synchronize the measurement\n-- between the two SMUs so set the built in delay to 0.\ndrain.measure.delay\t\t\t\t= 0\n\n-- Prepare the Reading Buffers\ndrain.nvbuffer1.clear()\ndrain.nvbuffer1.collecttimestamps= 1\ndrain.nvbuffer1.appendmode=1\ndrain.nvbuffer2.clear()\ndrain.nvbuffer2.collecttimestamps= 1\ndrain.nvbuffer2.appendmode=1\n--=============================\n-- End Channel B Settings", "-- Configure the Trigger Model\n--============================\n--Configurazione timer e trigger. Sono la parte essenziale dello script, dato che gestiscono i tempi di misura\ntrigger.clear()\n\n-- Timer 1 controls the pulse period, cioè la durata del gradino\ntimer_periodo.count\t\t\t= numPoints > 1 and numPoints - 1 or 1\ntimer_periodo.delay\t\t\t= pulsePeriod\n--il passthrough mi consente di ricevere l'interrupt quando il timer parte, ossia l'event id. \n--Mi servirà da stimolo per gli altri timer, che partiranno all'inizo del gradino\n-- definendo il momento della misura e la durata dell'impulso di alimentazione\ntimer_periodo.passthrough\t= true\n-- il timer 1 parte quando la drain, in questo caso, inizia la sweep: cioè entra nello stato armed\ntimer_periodo.stimulus\t\t= drain.trigger.ARMED_EVENT_ID \n\n-- Timer 2 controls the measurement. il timer 2 gestisce il ritardo di misura. scaduto quello, inizia la finestra di misura\ntimer_misura.count\t\t\t= 1\ntimer_misura.delay\t\t\t= measdelay\n-- il passthrough è false perchè l'interrupt lo produrre alla fine. \n-- Scaduto il delay di misura, inizia la finestra di misura\ntimer_misura.passthrough\t= false\n--il timer 1 grazie al passthrough mi fa partire il timer 2 all'inizio del gradino\ntimer_misura.stimulus\t\t= timer_periodo.EVENT_ID \n\n-- Timer 3 controls the pulse width\ntimer_larghezza_impulso.count\t\t\t= 1\ntimer_larghezza_impulso.delay\t\t\t= pulseWidth\n-- il passthrough è false perchè l'interrupt me lo produce alla fine, perchè \ntimer_larghezza_impulso.passthrough\t= false\n--il timer 1 grazie al passthrough mi fa partire il timer 3 all'inizio del gradino\ntimer_larghezza_impulso.stimulus\t\t= timer_periodo.EVENT_ID\n", "limitI=1\ngate.source.output\t\t\t\t= gate.OUTPUT_ON\ndrain.source.output\t\t\t\t= drain.OUTPUT_ON\n\n\nfor i=1,numSweep,1 do \n\n-- Configure gate Trigger Model for Sweep\n-- imposto un singolo valore di tensione, costante per tutta la durata della sweep.\n-- quindi quello che ottengo è la sweep di un singolo valore. il risultato è appunto una valore costante\n--in lua a differenza del linguaggio c/c++, il primo elemento di un array ha indice 1, non 0\n\nif source_gate==1 then-----------------------\ngate.trigger.source.listv({livello_gate[i]})\ngate.trigger.source.limiti\t\t= limiti_gate\nelse -------------------------------------------\ngate.trigger.source.listi({livello_gate[i]})\ngate.trigger.source.limitv\t\t= limiti_gate\nend--------------------------------------------\n\ngate.trigger.measure.action\t\t= gate.ASYNC\ngate.trigger.measure.iv(gate.nvbuffer1, gate.nvbuffer2)\n--fine impulso: se voglio una dc sweep, anzichè mandare in idle l'uscita, la tengo costante\ngate.trigger.endpulse.action\t= gate.SOURCE_HOLD\n-- endsweep mi dice cosa fare quando finisce l'operazione sweep\ngate.trigger.endsweep.action\t= gate.SOURCE_HOLD\ngate.trigger.arm.count = 1\ngate.trigger.count\t\t\t\t= 1\n-- arm sweep indica quanto sweep deve fare \ndrain.trigger.arm.stimulus\t\t= 0\n--dico quali timer attivanzo le azioni\n\n--event blender per la partenza\ntrigger.blender[1].orenable = true\ntrigger.blender[1].stimulus[1] = gate.trigger.ARMED_EVENT_ID\ntrigger.blender[1].stimulus[2] = drain.trigger.ARMED_EVENT_ID \n\n--dico quali stimoli/timer attivanzo le azioni\ngate.trigger.source.stimulus = trigger.blender[1].EVENT_ID \ngate.trigger.measure.stimulus\t= trigger.timer[2].EVENT_ID\n--gate.trigger.endpulse.stimulus\t= drain.trigger.SWEEP_COMPLETE_EVENT_ID\ngate.trigger.endpulse.stimulus\t= drain.trigger.IDLE_EVENT_ID\n\ngate.trigger.source.action\t\t= gate.ENABLE\n\n-- Configure drain Trigger Model for Sweep\n\nif source_drain==1 then------------------------\ndrain.trigger.source.linearv(start_drain, stop_drain, numPoints)\ndrain.trigger.source.limiti\t\t= limiti_drain\nelse---------------------------------------------\ndrain.trigger.source.lineari(start_drain, stop_drain, numPoints)\ndrain.trigger.source.limitv\t\t= limiti_drain\nend---------------------------------------------\ndrain.trigger.measure.action\t\t= drain.ENABLE\ndrain.trigger.measure.iv(drain.nvbuffer1, drain.nvbuffer2)\n--fine impulso: se voglio una dc sweep, anzichè mandare in idle l'uscita, la tengo costante\ndrain.trigger.endpulse.action\t= drain.SOURCE_HOLD \n-- endsweep mi dice cosa fare quando finisce l'operazione sweep\ndrain.trigger.endsweep.action\t= drain.SOURCE_HOLD\ndrain.trigger.arm.count = 1\n-- num punti sweep\ndrain.trigger.count\t\t\t\t= numPoints\n-- arm sweep indica quanto sweep deve fare\ndrain.trigger.arm.stimulus\t\t= 0\n--dico quali timer attivanzo le azioni\ndrain.trigger.source.stimulus\t= trigger.timer[1].EVENT_ID\ndrain.trigger.measure.stimulus\t= trigger.timer[2].EVENT_ID\ndrain.trigger.endpulse.stimulus\t= trigger.timer[3].EVENT_ID\ndrain.trigger.source.action\t\t= drain.ENABLE\n--==============================\n-- End Trigger Model Configuration\n\n-- Start the trigger model execution\ngate.trigger.initiate()\ndelay(0.05)\ndrain.trigger.initiate()\n\n-- Wait until the sweep has completed\nwaitcomplete()\n\n\n-- Configure gate Trigger Model for Sweep\n-- imposto un singolo valore di tensione, costante per tutta la durata della sweep.\n-- quindi quello che ottengo è la sweep di un singolo valore. il risultato è appunto una valore costante\nif source_gate==1 then-----------------------\ngate.trigger.source.listv({livello_gate[i]})\ngate.trigger.source.limiti\t\t= limiti_gate\nelse -------------------------------------------\ngate.trigger.source.listi({livello_gate[i]})\ngate.trigger.source.limitv\t\t= limiti_gate\nend--------------------------------------------\ngate.trigger.measure.action\t\t= gate.ASYNC\ngate.trigger.measure.iv(gate.nvbuffer1, gate.nvbuffer2)\n--fine impulso: se voglio una dc sweep, anzichè mandare in idle l'uscita, la tengo costante\ngate.trigger.endpulse.action\t= gate.SOURCE_HOLD\n-- endsweep mi dice cosa fare quando finisce l'operazione sweep\ngate.trigger.endsweep.action\t= gate.SOURCE_HOLD\ngate.trigger.arm.count = 1\ngate.trigger.count\t\t\t\t= 1\n-- arm sweep indica quanto sweep deve fare \ndrain.trigger.arm.stimulus\t\t= 0\n--dico quali timer attivanzo le azioni\n\n--event blender per la partenza\ntrigger.blender[1].orenable = true\ntrigger.blender[1].stimulus[1] = gate.trigger.ARMED_EVENT_ID\ntrigger.blender[1].stimulus[2] = drain.trigger.ARMED_EVENT_ID \n\n--dico quali stimoli/timer attivanzo le azioni\ngate.trigger.source.stimulus = trigger.blender[1].EVENT_ID \ngate.trigger.measure.stimulus\t= trigger.timer[2].EVENT_ID\n--gate.trigger.endpulse.stimulus\t= drain.trigger.SWEEP_COMPLETE_EVENT_ID\ngate.trigger.endpulse.stimulus\t= drain.trigger.IDLE_EVENT_ID\n\n--gate.trigger.source.action\t\t= gate.ENABLE\n\n-- Configure drain Trigger Model for Sweep\n\nif source_drain==1 then------------------------\ndrain.trigger.source.linearv(stop_drain, start_drain, numPoints)\ndrain.trigger.source.limiti\t\t= limiti_drain\nelse---------------------------------------------\ndrain.trigger.source.lineari(stop_drain, start_drain, numPoints)\ndrain.trigger.source.limitv\t\t= limiti_drain\nend---------------------------------------------\ndrain.trigger.measure.action\t\t= drain.ENABLE\ndrain.trigger.measure.iv(drain.nvbuffer1, drain.nvbuffer2)\n--fine impulso: se voglio una dc sweep, anzichè mandare in idle l'uscita, la tengo costante\ndrain.trigger.endpulse.action\t= drain.SOURCE_HOLD \n-- endsweep mi dice cosa fare quando finisce l'operazione sweep\ndrain.trigger.endsweep.action\t= drain.SOURCE_HOLD\ndrain.trigger.arm.count = 1\n-- num punti sweep\ndrain.trigger.count\t\t\t\t= numPoints\n-- arm sweep indica quanto sweep deve fare\ndrain.trigger.arm.stimulus\t\t= 0\n--dico quali timer attivanzo le azioni\ndrain.trigger.source.stimulus\t= trigger.timer[1].EVENT_ID\ndrain.trigger.measure.stimulus\t= trigger.timer[2].EVENT_ID\ndrain.trigger.endpulse.stimulus\t= trigger.timer[3].EVENT_ID\n--drain.trigger.source.action\t\t= drain.ENABLE\n--==============================\n-- End Trigger Model Configuration\n\n-- Start the trigger model execution\ngate.trigger.initiate()\n--delay(0.05)\ndrain.trigger.initiate()\nwaitcomplete()\nend\n\ndrain.source.output\t\t\t\t= drain.OUTPUT_OFF\ndelay(0.05)\ngate.source.output\t\t\t\t= gate.OUTPUT_OFF\n\n--printbuffer(1, numPoints, gate.nvbuffer2.readings)\n--printbuffer(1, numPoints, gate.nvbuffer1.readings)\n--printbuffer(1, numPoints, gate.nvbuffer1.timestamps)\n\n--printbuffer(1, numPoints, drain.nvbuffer2.readings)\n--printbuffer(1, numPoints, drain.nvbuffer1.readings)\n--printbuffer(1, numPoints, drain.nvbuffer1.timestamps)" ("write buffer")) -> (w139:string)
                n22 = Multiply(x=w137, y=2) -> (x*y=w138:i32)
              }
            }
            n23 = Format Into String(format string=w105, w104, w103, w102, w101, w100, w99, w98, w97, w96, w95, w94, w93, w92, w91, w88, w87, w89, w90, w85, w84, w81, w80) -> (resulting string=w122:string)  [unwired: 2 in, 1 out]
            n24 = call <instrlib>:"Create Script.vi"("Auto Run (F: Disable)"=TRUE, "error in (no error)"=w123, "Source Code"=w122, "Script Variable"="myScript", "VISA resource name"=w124) -> ("error out"=w118:errorcluster, "VISA resource name out"=w119:refnum<visa-resource-name>)  [unwired: 5 in]
            n25 = call "lettura_dati.vi"("error in (no error)"=w118, "Source Measure Unit Channel (0: Channel A)"=w115, "End Index (1)"=w82, "VISA resource name"=w119) -> ("error out"=w116:errorcluster, "CORRENTE"=→"SMUB-CORRENTE":dbl[], "TENSIONE"=→"SMUB-TENSIONE":dbl[], "VISA resource name out"=w117:refnum<visa-resource-name>, "TEMPI"=→"SMUB-TEMPI":dbl[])  [unwired: 3 in]
            n26 = call "lettura_dati.vi"("error in (no error)"=w116, "Source Measure Unit Channel (0: Channel A)"=w112, "End Index (1)"=w82, "VISA resource name"=w117) -> ("error out"=w113:errorcluster, "CORRENTE"=→"SMUA-CORRENTE":dbl[], "TENSIONE"=→"SMUA-TENSIONE":dbl[], "VISA resource name out"=w114:refnum<visa-resource-name>, "TEMPI"=→"SMUA-TEMPI":dbl[])  [unwired: 3 in]
          }
        }
      }
    }
    frame #3 {
      n27 = call <instrlib>:"Close.vi"("error in (no error)"=w146, "VISA resource name"=w147) -> ()  [unwired: 9 in, 1 out]
    }
  }
